vi "myfourthvi.vi"() -> ()   [LabVIEW 2019]
panel:
  out "size(s)":i32[](array[numeric])
  out "appended array":i32[](array[numeric])
  in  "Colors":T1
  in  "path to PNG file":path
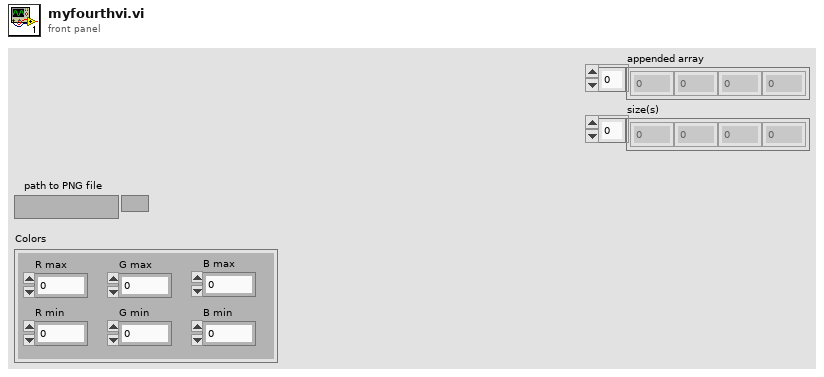
[diagram p1: front panel]
types:
  T1 = cluster{"R max":dbl, "G max":dbl, "B max":dbl, "R min":dbl, "G min":dbl, "B min":dbl}
  T2 = typedef "imagedata.ctl" = cluster{"image type":i32, "image depth":i32, "image":u8[], "mask":u8[], "colors":u32[], "Rectangle":cluster{"left":i16, "top":i16, "right":i16, "bottom":i16}}
  T3 = cluster{"[0]":i32, "[1]":i32, "[2]":i32, "[3]":i32, "[4]":i32, "[5]":i32, "[6]":i32, "[7]":i32, "[8]":i32}
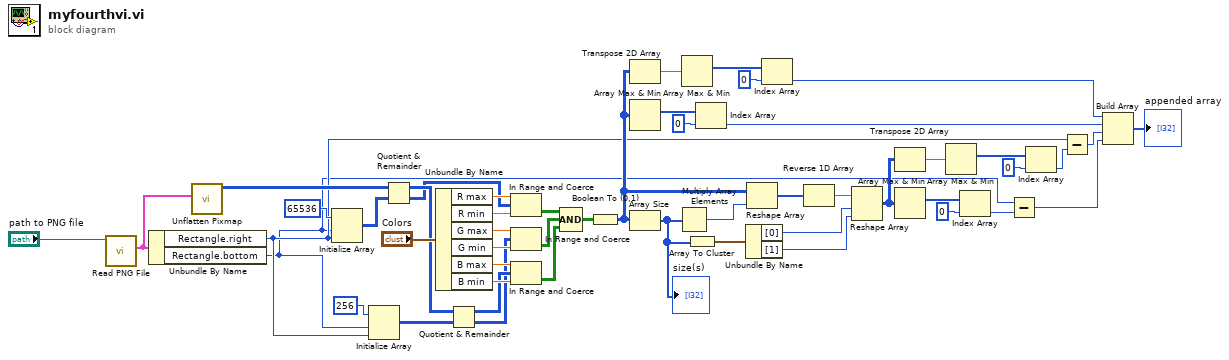
[diagram p0: block diagram]
diagram:
  n1 = call <vilib>:"Read PNG File.vi"("path to PNG file"="path to PNG file") -> ("image data"=w48:T2)  [unwired: 8 in, 2 out]
  n2 = Unbundle By Name(w48) -> ("Rectangle.right"=w6:i16, "Rectangle.bottom"=w5:i16)
  n3 = call <vilib>:"Unflatten Pixmap.vi"("image data"=w48) -> ("24-bit pixmap"=w30:u32[][])  [unwired: 4 in, 6 out]
  n4 = Initialize Array(65536, w5, w6) -> (w31:i32[][])
  n5 = Initialize Array(256, w5, w6) -> (w32:i32[][])
  n6 = Quotient & Remainder(x=w30, y=w31) -> (x-y*floor(x/y)=w41:u32[][], floor(x/y)=w38:u32[][])
  n7 = Unbundle By Name("Colors") -> ("R max"=w47:dbl, "R min"=w46:dbl, "G max"=w45:dbl, "G min"=w44:dbl, "B max"=w43:dbl, "B min"=w42:dbl)
  n8 = Quotient & Remainder(x=w41, y=w32) -> (x-y*floor(x/y)=w40:u32[][], floor(x/y)=w39:u32[][])
  n9 = In Range and Coerce(upper limit=w47, x=w38, lower limit=w46) -> (In Range?=w37:bool[][])  [unwired: 1 out]
  n10 = In Range and Coerce(upper limit=w45, x=w39, lower limit=w44) -> (In Range?=w36:bool[][])  [unwired: 1 out]
  n11 = In Range and Coerce(upper limit=w43, x=w40, lower limit=w42) -> (In Range?=w35:bool[][])  [unwired: 1 out]
  n12 = Compound Arithmetic op=AND(w37, w36, w35) -> (w29:bool[][])
  n13 = Boolean To (0,1)(Boolean=w29) -> (0, 1=w20:i16[][])
  n14 = Transpose 2D Array(2D array=w20) -> (transposed array=w28:i16[][])
  n15 = Array Max & Min(array=w20) -> (max index (indices)=w27:i32[])  [unwired: 3 out]
  n16 = Array Size(array=w20) -> (size(s)=w17:i32[])
  "size(s)" <- w17
  n17 = Multiply Array Elements(1:w17) -> (0:w16:i32)
  n18 = Array Max & Min(array=w28) -> (max index (indices)=w25:i32[])  [unwired: 3 out]
  n19 = Array To Cluster(array=w17) -> (cluster=w15:T3)
  n20 = Index Array(array=w27, index=0) -> (element=w22:i32)
  n21 = Unbundle By Name(w15) -> ("[0]"=w14:i32, "[1]"=w13:i32)
  n22 = Reshape Array(w20, w16) -> (w19:i16[])
  n23 = Index Array(array=w25, index=0) -> (element=w23:i32)
  n24 = Reverse 1D Array(array=w19) -> (reversed array=w18:i16[])
  n25 = Reshape Array(w18, w14, w13) -> (w7:i16[][])
  n26 = Transpose 2D Array(2D array=w7) -> (transposed array=w12:i16[][])
  n27 = Array Max & Min(array=w7) -> (max index (indices)=w11:i32[])  [unwired: 3 out]
  n28 = Array Max & Min(array=w12) -> (max index (indices)=w9:i32[])  [unwired: 3 out]
  n29 = Index Array(array=w11, index=0) -> (element=w2:i32)
  n30 = Subtract(x=w5, y=w2) -> (x-y=w1:i32)
  n31 = Index Array(array=w9, index=0) -> (element=w4:i32)
  n32 = Subtract(x=w6, y=w4) -> (x-y=w3:i32)
  n33 = Build Array(w23, w22, w3, w1) -> (→"appended array":i32[])
